vi "DAQ - Initialize.vi"(8 "error in (no error)":errorcluster, 11 "DAQ":tag) -> (0 "error out":errorcluster)   [LabVIEW 2020]
uses:
  DAQ Globals.vi
  <vilib>/DAQmx/create/channels.llb/DAQmx Create Channel (AI-Voltage-Basic).vi
  <vilib>/DAQmx/configure/timing.llb/DAQmx Timing (Sample Clock).vi
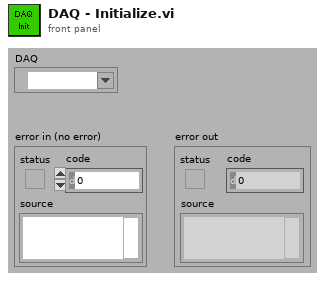
[diagram p1: front panel]
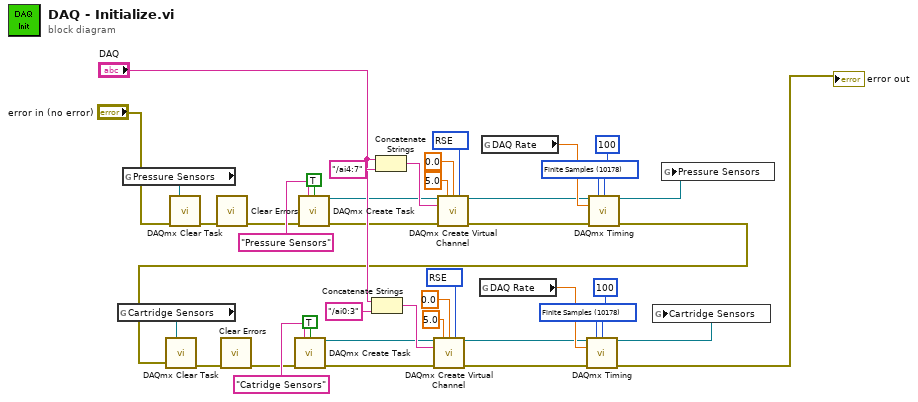
[diagram p0: block diagram]
diagram:
  w4 = 10083 items=["Default"=-1, "RSE"=10083, "NRSE"=10078, "Differential"=10106, "Pseudodifferential"=12529] ("input terminal configuration")
  w5 = 10083 items=["Default"=-1, "RSE"=10083, "NRSE"=10078, "Differential"=10106, "Pseudodifferential"=12529] ("input terminal configuration")
  w11 = 10178 items=["Finite Samples"=10178, "Continuous Samples"=10123, "Hardware Timed Single Point"=12522] ("sample mode")
  w20 = 10178 items=["Finite Samples"=10178, "Continuous Samples"=10123, "Hardware Timed Single Point"=12522] ("sample mode")
  n1 = global read "DAQ Globals.vi" "Cartridge Sensors"() -> (w29:refnum<k21>)
  n2 = global read "DAQ Globals.vi" "Pressure Sensors"() -> (w39:refnum<k21>)
  n3 = call <vilib>:"DAQmx Clear Task.vi"("task in"=w39, "error in"="error in (no error)") -> ("error out"=w36:errorcluster)  [unwired: 13 in]
  n4 = call <vilib>:"Clear Errors.vi"("error in (no error)"=w36) -> ("error out"=w3:errorcluster)  [unwired: 5 in, 1 out]
  n5 = call <vilib>:"DAQmx Create Task.vi"("new task name"="Pressure Sensors", "auto cleanup"=TRUE, "error in"=w3) -> ("task out"=w23:refnum<k21>, "error out"=w22:errorcluster)  [unwired: 11 in]
  n6 = Concatenate Strings("DAQ", "/ai0:3" ("new task name")) -> (w33:string)
  n7 = Concatenate Strings("DAQ", "/ai4:7" ("new task name")) -> (w34:string)
  n8 = call-poly <vilib>:"DAQmx Create Virtual Channel.vi"("task in"=w23, "maximum value"=5.0, "minimum value"=0.0, "input terminal configuration"=w5, "physical channels"=w34, "error in"=w22) -> ("task out"=w18:refnum<k21>, "error out"=w17:errorcluster)  [unwired: 8 in]
  n9 = global read "DAQ Globals.vi" "DAQ Rate"() -> (w10:dbl)
  n10 = global read "DAQ Globals.vi" "DAQ Rate"() -> (w21:dbl)
  n11 = call-poly <vilib>:"DAQmx Timing.vi"("task/channels in"=w18, "sample mode"=w20, "samples per channel"=100, "rate"=w21, "error in"=w17) -> ("task out"=w16:refnum<k21>, "error out"=w15:errorcluster)  [unwired: 9 in]
  n12 = call <vilib>:"DAQmx Clear Task.vi"("task in"=w29, "error in"=w15) -> ("error out"=w2:errorcluster)  [unwired: 13 in]
  n13 = call <vilib>:"Clear Errors.vi"("error in (no error)"=w2) -> ("error out"=w1:errorcluster)  [unwired: 5 in, 1 out]
  n14 = call <vilib>:"DAQmx Create Task.vi"("new task name"="Catridge Sensors", "auto cleanup"=TRUE, "error in"=w1) -> ("task out"=w14:refnum<k21>, "error out"=w13:errorcluster)  [unwired: 11 in]
  n15 = call-poly <vilib>:"DAQmx Create Virtual Channel.vi"("task in"=w14, "maximum value"=5.0, "minimum value"=0.0, "input terminal configuration"=w4, "physical channels"=w33, "error in"=w13) -> ("task out"=w9:refnum<k21>, "error out"=w8:errorcluster)  [unwired: 8 in]
  n16 = call-poly <vilib>:"DAQmx Timing.vi"("task/channels in"=w9, "sample mode"=w11, "samples per channel"=100, "rate"=w10, "error in"=w8) -> ("task out"=w7:refnum<k21>, "error out"=→"error out":errorcluster)  [unwired: 9 in]
  n17 = global write "DAQ Globals.vi" "Cartridge Sensors"(w7) -> ()
  n18 = global write "DAQ Globals.vi" "Pressure Sensors"(w16) -> ()
